vi "Bytes at port more than X.vi"(3 "error IO":errorcluster, 4 "X":u32, 5 "port in":refnum<visa-resource-name>) -> (0 "error out":errorcluster, 1 "Bytes at port > X":bool, 2 "port out":refnum<visa-resource-name>)   [LabVIEW 2013]
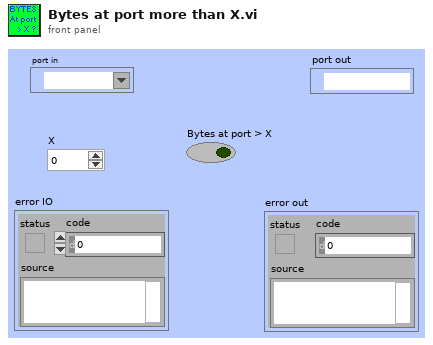
[diagram p1: front panel]
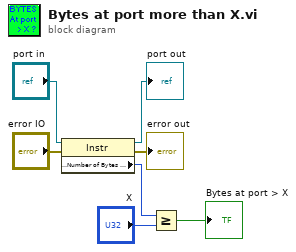
[diagram p0: block diagram]
diagram:
  n1 = property class="Instr"(reference="port in", error in="error IO") -> (reference out=→"port out":refnum<visa-resource-name>, error out=→"error out":errorcluster, "Serial Settings:Number of Bytes at Serial Port"=w2:u32)
  n2 = Greater Or Equal?(x=w2, y="X") -> (x >= y?=→"Bytes at port > X":bool)
